vi "Calibration Cal Execute RF Test Get Default LSL.vi"(8 "error in (no error)":errorcluster, 11 "Template Tx Test in":refnum<class "niDTS Calibration Cal Execute RF Test.lvclass">) -> (0 "error out":errorcluster, 2 "Default LSL":T1, 3 "Template Tx Test out":refnum<class "niDTS Calibration Cal Execute RF Test.lvclass">)   [LabVIEW 2015, in "niDTS Utilities.lvlib" / "niDTS Calibration Cal Execute RF Test.lvclass"]
uses:
  niDTS Calibration Cal Execute RF Test.lvclass
  Includes/niDTS Calibration Cal Execute RF Test INC Results.ctl
  niDTS Utilities.lvlib
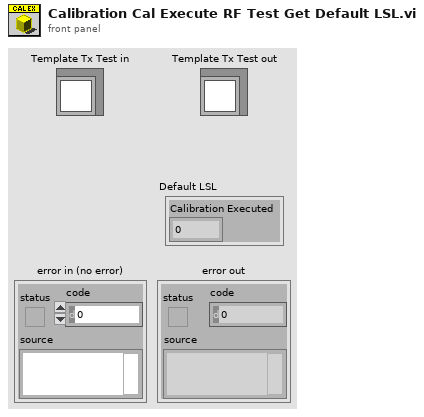
[diagram p1: front panel]
types:
  T1 = typedef "niDTS Utilities.lvlib/niDTS Calibration Cal Execute RF Test INC Results.ctl" = cluster{"Calibration Executed":u8}
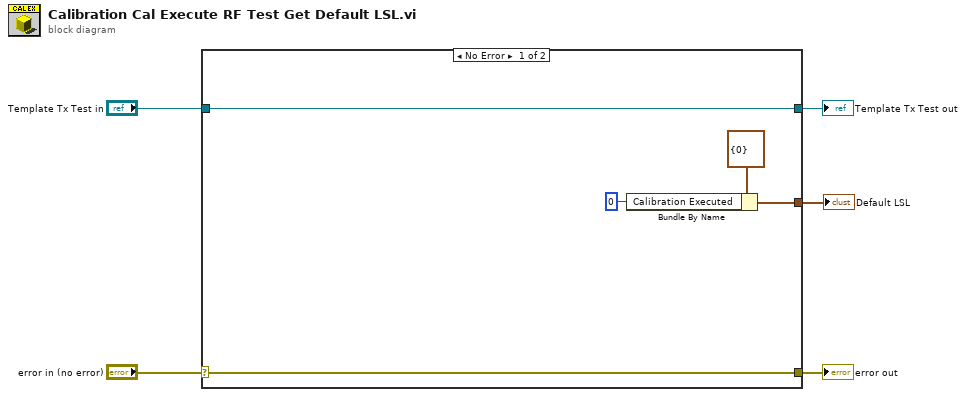
[diagram p0: block diagram]
diagram:
  n1 = case shown="No Error" "error in (no error)" {
    selector: "error in (no error)" -> [w10 w12]
    tunnel: [w10 w12] -> w4
    tunnel: [w9 w11] -> w2
    tunnel: "Template Tx Test in" -> [w9 w11]
    tunnel: [w7 _] -> w1
    frame No Error {
      n2 = Bundle By Name(cluster=T1 {"Calibration Executed"=0} ("Default LSL"), "Calibration Executed"=u8 0) -> (w7:T1)
    }
    frame Error {
    }
  }
  "error out" <- w4
  "Template Tx Test out" <- w2
  "Default LSL" <- w1
